vi "Add Frame to Image.vi"(6 "Option":T1={"pen"={"Width"=1, "Style"=enum."Solid"}, "color(black)"=0}, 8 "错误输入":errorcluster, 9 "Frame?":bool, 10 "image data":T2 caption="图像数据", 11 "Picture in":picture) -> (0 "错误输出":errorcluster, 3 "Picture out":picture)   [LabVIEW 2012, in "Picture Box Tools.lvlib"]
uses:
  Picture Box Tools.lvlib
  <vilib>/picture/picture.llb/imagedata.ctl
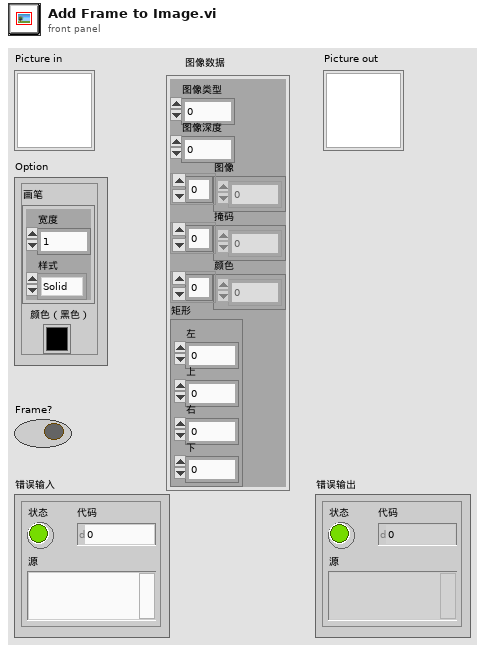
[diagram p1: front panel]
types:
  T1 = cluster{"pen":cluster{"Width":i16, "Style":enum32{"Solid", "Dash", "Dot", "DashDot", "DashDotDot"}}, "color(black)":u32}
  T2 = typedef "imagedata.ctl" = cluster{"image type":i32, "image depth":i32, "image":u8[], "mask":u8[], "colors":u32[], "Rectangle":cluster{"left":i16, "top":i16, "right":i16, "bottom":i16}}
  T3 = cluster{"Width":i16, "Style":enum32{"Solid", "Dash", "Dot", "DashDot", "DashDotDot"}}
  T4 = cluster{"left":i16, "top":i16, "right":i16, "bottom":i16}
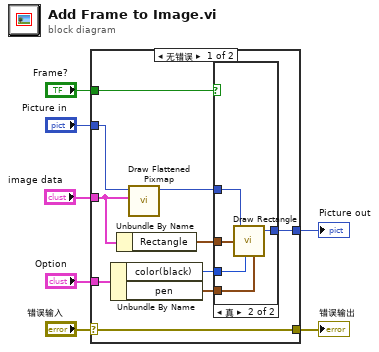
[diagram p0: block diagram]
diagram:
  n1 = case shown="无错误" "错误输入" {
    selector: "错误输入" -> [w12 w25]
    tunnel: [w15 w24] -> w7
    tunnel: [w12 w25] -> w5
    tunnel: "Picture in" -> [w11 w24]
    tunnel: "image data" -> [w10 _]
    tunnel: "Option" -> [w9 _]
    tunnel: "Frame?" -> [w8 _]
    frame No Error {
      n2 = Unbundle By Name(w9) -> ("color(black)"=w13:u32, "pen"=w14:T3)
      n3 = Unbundle By Name(w10) -> ("Rectangle"=w16:T4)
      n4 = call <vilib>:"Draw Flattened Pixmap.vi"("image data"=w10, "picture"=w11) -> ("new picture"=w17:picture)  [unwired: 7 in]
      n5 = case shown="真" w8 {
        tunnel: w17 -> [w18 w23]
        tunnel: w16 -> [_ w22]
        tunnel: [w18 w21] -> w15
        tunnel: w14 -> [_ w20]
        tunnel: w13 -> [_ w19]
        frame False {
        }
        frame True {
          n6 = call <vilib>:"Draw Rectangle.vi"("picture"=w23, "rect"=w22, "color(black)"=w19, "pen"=w20) -> ("new picture"=w21:picture)  [unwired: 5 in]
        }
      }
    }
    frame Error {
    }
  }
  "Picture out" <- w7
  "错误输出" <- w5
